vi "Sequence Update Table for Spartan 6.0.vi"(8 "error in (no error)":errorcluster, 11 "Connection Refnum":T1) -> (0 "error out":errorcluster, 3 "Connection Refnum":T1)   [LabVIEW 2011]
uses:
  SI.LIB/ODBC/SQL Controls/Connection Refnum.ctl
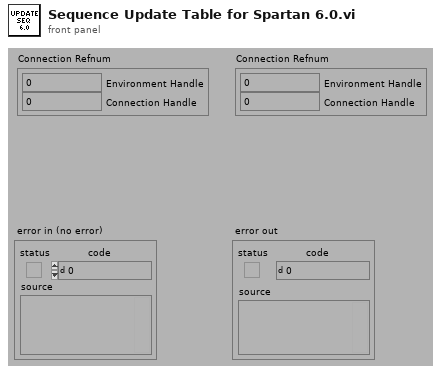
[diagram p1: front panel]
types:
  T1 = typedef "Connection Refnum.ctl" = cluster{"Environment Handle":i32, "Connection Handle":i32}
  T2 = typedef "Statement Refnum.ctl" = cluster{"Statement Handle":i32, "Parameter Number":u16}
  T3 = typedef "Sequence Record.ctl" = cluster{"ixSequence":i32, "sxSequenceId":string, "sDescription":string, "sCreator":string, "tCreationDate":timestamp, "sModifier":string, "tModifiedDate":timestamp, "fApproved":bool, "fSpartanSetsSN":bool, "fOverwriteData":bool, "fStopOnFail":bool, "fDisableQuickMode":bool, "fPartialExecution":bool, "fAutoNextItem":bool, "fDoNotPrintOnFail":bool}
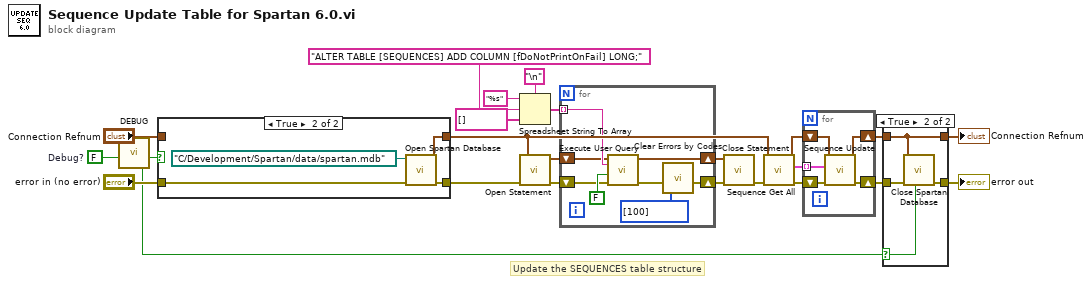
[diagram p0: block diagram]
diagram:
  w10 = FALSE  # Debug?
  # "Update the SEQUENCES table structure"
  n1 = call "DEBUG.vi"("Dev DEBUG? (f)"=w10) -> ("DEBUG?"=w9:bool)  [unwired: 1 in, 5 out]
  n2 = case shown="True" w9 {
    tunnel: "Connection Refnum" -> [w25 _]
    tunnel: "error in (no error)" -> [w24 w29]
    tunnel: [w24 w28] -> w11
    tunnel: [w25 w27] -> w4
    frame False {
    }
    frame True {
      n3 = call "Open Spartan Database.vi"("error in (no error)"=w29, "DB Path (empty - use default)"=path "C:/Development/Spartan/data/spartan.mdb" ("DB Path")) -> ("error out"=w28:errorcluster, "Connection Refnum"=w27:T1)  [unwired: 1 in, 7 out]
    }
  }
  n4 = Spreadsheet String To Array(delimiter (Tab)="\n", format string="%s", spreadsheet string="ALTER TABLE [SEQUENCES] ADD COLUMN [fDoNotPrintOnFail] LONG;" ("User Query"), array type (2D Dbl)=string[] []) -> (array=w22:string[])
  n5 = call "Open Statement.vi"("error in (no error)"=w11, "Connection Refnum"=w4) -> ("error out"=w19:errorcluster, "Statement Refnum"=w18:T2)  [unwired: 4 out]
  n6 = for {
    shift-right: [w30] -> w17
    shift-left: w19 -> [w34]
    tunnel: w22 -> [w36] mode=indexing
    shift-right: [w33] -> w16
    shift-left: w18 -> [w35]
    n7 = call "Execute User Query.vi"("error in (no error)"=w34, "Return Data? (f)"=FALSE, "User Query"=w36, "Statement Refnum"=w35) -> ("error out"=w31:errorcluster, "Statement Refnum"=w33:T2)  [unwired: 2 out]
    n8 = call "Clear Errors by Codes.vi"("Error Codes\nto Clear (Empty)"=i32[] [100] ("Error Codes\nto Clear (Empty)"), "error in (no error)"=w31) -> ("error out"=w30:errorcluster)  [unwired: 5 out]
  }
  n9 = call "Close Statement.vi"("error in (no error)"=w17, "Statement Refnum"=w16) -> ("error out"=w6:errorcluster)  [unwired: 5 out]
  n10 = call "Sequence Get All.vi"("error in (no error)"=w6, "Connection Refnum"=w4) -> ("error out"=w7:errorcluster, "Sequence Records"=w1:T3[], "Connection Refnum"=w3:T1)  [unwired: 5 in, 2 out]
  n11 = for {
    shift-right: [w39] -> w2
    shift-left: w3 -> [w40]
    tunnel: w1 -> [w38] mode=indexing
    shift-right: [w41] -> w5
    shift-left: w7 -> [w42]
    n12 = call "Sequence Update.vi"("error in (no error)"=w42, "Sequence Record"=w38, "Connection Refnum"=w40) -> ("error out"=w41:errorcluster, "Connection Refnum"=w39:T1)  [unwired: 7 in]
  }
  n13 = case shown="True" w9 {
    selector: w9 -> [_ w45]
    tunnel: w5 -> [w44 w48]
    tunnel: w2 -> [w43 w46]
    tunnel: [w43 w46] -> w15
    tunnel: [w44 w47] -> w14
    frame False {
    }
    frame True {
      n14 = call "Close Spartan Database.vi"("Force Close? (f)"=w45, "error in (no error)"=w48, "Connection Refnum"=w46) -> ("error out"=w47:errorcluster)  [unwired: 2 in, 6 out]
    }
  }
  "error out" <- w14
  "Connection Refnum" <- w15
